vi "ev c change.vi"(8 "error in (no error)":errorcluster, 11 "IDE simple in":refnum<class "LF2R IDE.lvclass">) -> (0 "error out":errorcluster, 3 "IDE simple out":refnum<class "LF2R IDE.lvclass">)   [LabVIEW 2018, in "LF2R IDE.lvlib" / "LF2R IDE.lvclass"]
uses:
  LF2R IDE.lvclass
  LF2R IDE.lvclass/LF2R IDE.ctl
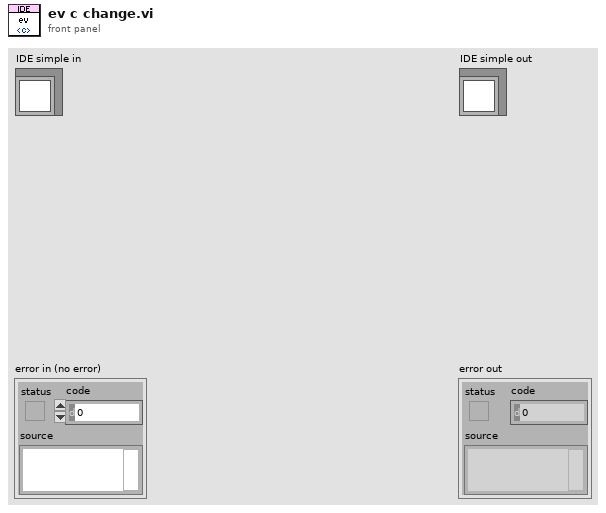
[diagram p1: front panel]
types:
  T1 = typedef "Data Parser.lvclass/frame c data.ctl" = cluster{"kind":string, "x":string, "y":string, "injury":string, "cover":string, "vaction":string, "aaction":string, "taction":string, "hurtable":string, "decrease":string, "fronthurtact":string, "backhurtact":string, "dircontrol":string, "throwvx":string, "throwvy":string, "throwvz":string, "throwinjury":string}
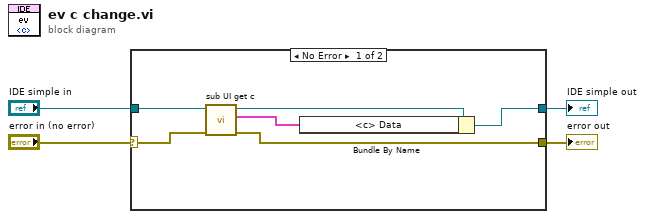
[diagram p0: block diagram]
diagram:
  n1 = case shown="No Error" "error in (no error)" {
    selector: "error in (no error)" -> [w9 w12]
    tunnel: [w6 w12] -> w3
    tunnel: [w5 w11] -> w1
    tunnel: "IDE simple in" -> [w10 w11]
    frame No Error {
      n2 = call "sub UI get c.vi"("error in (no error)"=w9, "IDE simple in"=w10) -> ("error out"=w6:errorcluster, "<c> data"=w7:T1, "IDE simple out"=w8:refnum<class "LF2R IDE.lvclass">)  [unwired: 7 in]
      n3 = Bundle By Name(cluster=w8, "<c> Data"=w7) -> (w5:refnum<class "LF2R IDE.lvclass">)
    }
    frame Error {
    }
  }
  "error out" <- w3
  "IDE simple out" <- w1
